vi "TaborSkipThrough.vi"(9 "Voltage Steps":sgl[](array[numeric])=[100.0] format="%_3g", 10 "Burst Ct":i8[](array[numeric])=[1, 3, 5, 10, 20], 11 "Time Step (ms)":i64=5000) -> ()   [LabVIEW 2022 SP3]
uses:
  Motion Controllers/-MotionRoutines/MotionGlobals.vi
  <vilib>/Platform/TimedLoop/XDataNode/XDataNode.xnode
  <vilib>/Platform/TimedLoop/XDataNode/nitl_modes.ctl
  <vilib>/Platform/TimedLoop/XDataNode/XDNodeRunTimeDep.lvlib
  <vilib>/Platform/TimedLoop/XDataNode/wakeup.ctl
  <vilib>/Platform/TimedLoop/XDataNode/timing_clust.ctl
panel:
  out "Current Voltage (mV)":sgl
  out "Current Burst":i8
  # "Inputs (don't change once running)"
  # "Current Values"
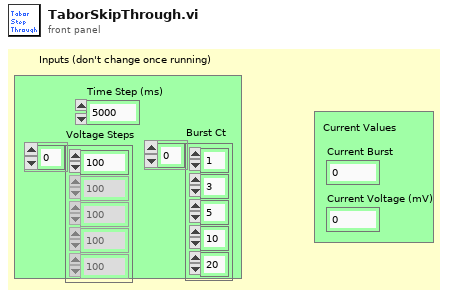
[diagram p1: front panel]
types:
  T1 = typedef "XDNodeRunTimeDep.lvlib/timing_clust.ctl" = cluster{"Expected End [f-1]":u64, "Actual End [f-1]":u64, "Finished Late? [f-1]":bool, "Expected End [i-1]":u64, "Actual End [i-1]":u64, "Finished Late? [i-1]":bool, "Expected Start [i]":u64, "Actual Start [i]":u64, "Expected Start [f]":u64, "Actual Start [f]":u64, "Source Name":string, "Structure Name":string, "Period":i64, "Deadline":i64, "Offset":i64, "Start":i64, "Priority":i32, "Timeout":i32, "Mode":T2, "Wakeup Reason":T3, "Error":errorcluster, "Source Type":string, "Secondary Source Type":string, "Global End Time":u64, "Global Start Time":u64, "Frame Duration":u64, "Iteration Duration":u64, "Assigned CPU":i32, "I/O Scan Engine Mode":u32}
  T2 = typedef "XDNodeRunTimeDep.lvlib/nitl_modes.ctl" = enum32{"No Change", "Process missed periods, maintain original phase", "Discard missed periods, maintain original phase", "Process missed periods, ignore original phase", "Discard missed periods, ignore original phase"}
  T3 = typedef "XDNodeRunTimeDep.lvlib/wakeup.ctl" = enum32{"Normal", "Aborted", "Asynchronous wakeup", "Timing source error", "Timed loop error", "Timeout"}
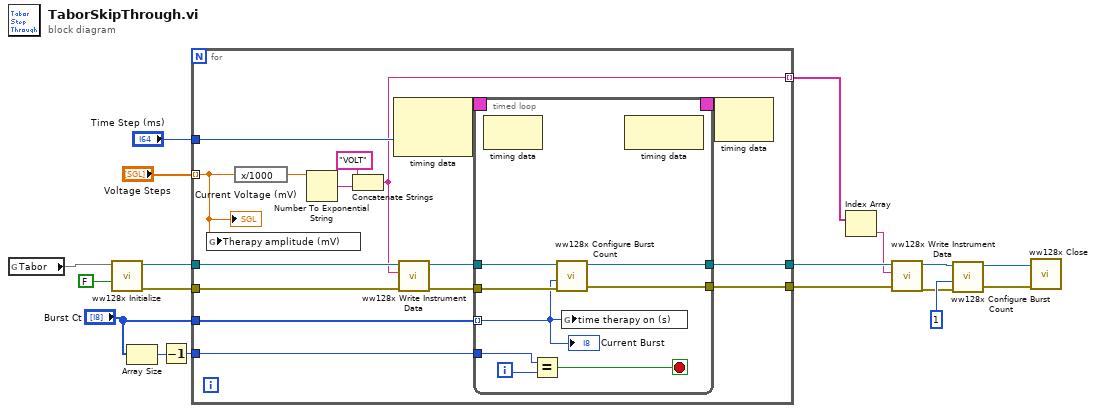
[diagram p0: block diagram]
diagram:
  n1 = global read "MotionGlobals.vi" "Tabor"() -> (w17)
  n2 = call <instrlib>:"ww128x Initialize.vi"("reset device (Yes)"=FALSE ("reset device"), "resource name"=w17) -> ("error out"=w15:errorcluster, "instrument handle out"=w16:refnum<k15>)  [unwired: 2 in, 6 out]
  n3 = Array Size(array="Burst Ct") -> (size(s)=w11:i32)
  n4 = Decrement(x=w11) -> (x-1=w10:i32)
  n5 = for {
    tunnel: w16 -> [w32]
    tunnel: w15 -> [w31]
    tunnel: "Voltage Steps" -> [w29] mode=indexing
    tunnel: "Burst Ct" -> [w21]
    tunnel: "Time Step (ms)" -> [w24]
    tunnel: [w23] -> w5
    tunnel: [w22] -> w4
    tunnel: w10 -> [w20]
    tunnel: [w19] -> w6 mode=indexing
    n6 = global write "MotionGlobals.vi" "Therapy amplitude (mV)"(w29) -> ()
    n7 = expression code="x/1000"(w29) -> (w30:sgl)
    n8 = Number To Exponential String(number=w30) -> (E-format string=w34:string)  [unwired: 3 out]
    n9 = Concatenate Strings("VOLT" ("string"), w34) -> (w19:string)
    n10 = node-c288(w24) -> (w28:T1)  [unwired: 1 in]
    n11 = call <instrlib>:"ww128x Write Instrument Data.vi"("error in (no error)"=w31, "write buffer"=w19, "instrument handle"=w32) -> ("error out"=w25:errorcluster, "instrument handle out"=w26:refnum<k15>)  [unwired: 7 out]
    n12 = timed-loop {
      timing: w28 -> [_]
      timing-out: [_] -> w27
      tunnel: w26 -> [w42]
      tunnel: w25 -> [w41]
      tunnel: w21 -> [w40] mode=indexing
      tunnel: [w39] -> w23
      tunnel: [w38] -> w22
      tunnel: w20 -> [w36]
      i -> [w37]
      stop <- w35 stop-if-true
      n13 = node-c288() -> ()  [unwired: 1 in, 1 out]
      n14 = Equal?(x=w36, y=w37) -> (x = y?=w35:bool)
      n15 = call <instrlib>:"ww128x Configure Burst Count.vi"("error in (no error)"=w41, "burst count (2)"=w40, "instrument handle"=w42) -> ("error out"=w38:errorcluster, "instrument handle out"=w39:refnum<k15>)  [unwired: 1 in, 6 out]
      n16 = global write "MotionGlobals.vi" "time therapy on (s)"(w40) -> ()
      n17 = node-c288() -> ()  [unwired: 1 in, 1 out]
      "Current Burst" <- w40
    }
    n18 = node-c288(w27) -> ()  [unwired: 1 out]
    "Current Voltage (mV)" <- w29
  }
  n19 = Index Array(array=w6) -> (element=w3:string)  [unwired: 1 in]
  n20 = call <instrlib>:"ww128x Write Instrument Data.vi"("error in (no error)"=w4, "write buffer"=w3, "instrument handle"=w5) -> ("error out"=w1:errorcluster, "instrument handle out"=w2:refnum<k15>)  [unwired: 7 out]
  n21 = call <instrlib>:"ww128x Configure Burst Count.vi"("error in (no error)"=w1, "burst count (2)"=1, "instrument handle"=w2) -> ("error out"=w8:errorcluster, "instrument handle out"=w9:refnum<k15>)  [unwired: 1 in, 6 out]
  n22 = call <instrlib>:"ww128x Close.vi"("error in (no error)"=w8, "instrument handle"=w9) -> ()  [unwired: 9 in, 1 out]
